vi "Create EQE Data Folder and File Path.vi"(6 "Skip cell?":bool, 7 "Date array":string[](array[string]), 9 "Cell details cluster":T1={"Cell Position"=16, "Cell Label"="", "Pixel to measure"=0, "Area (cm^2)"=0.126, "Variable"="", "Variable value"="", "Scan settings in queue"=0, "Light or dark"="", "Measurement Type"=""} {"Pixel to measure" items=["All", "1", "2", "3", "4", "5", "6", "7", "8"]}, 10 "Experiment Indicator":string, 11 "username":string) -> (1 "EQE data file path string":string, 2 "EQE data file path":path, 3 "EQE Data Output Folder":path)   [LabVIEW 2011]
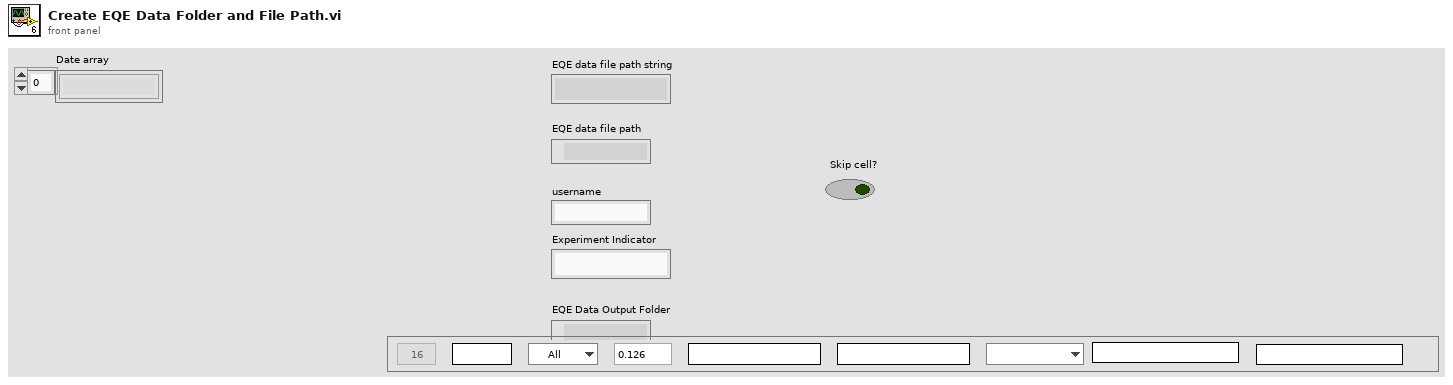
[diagram p1: front panel]
types:
  T1 = cluster{"Cell Position":i32, "Cell Label":string, "Pixel to measure":u16, "Area (cm^2)":dbl, "Variable":string, "Variable value":string, "Scan settings in queue":u16, "Light or dark":string, "Measurement Type":string}
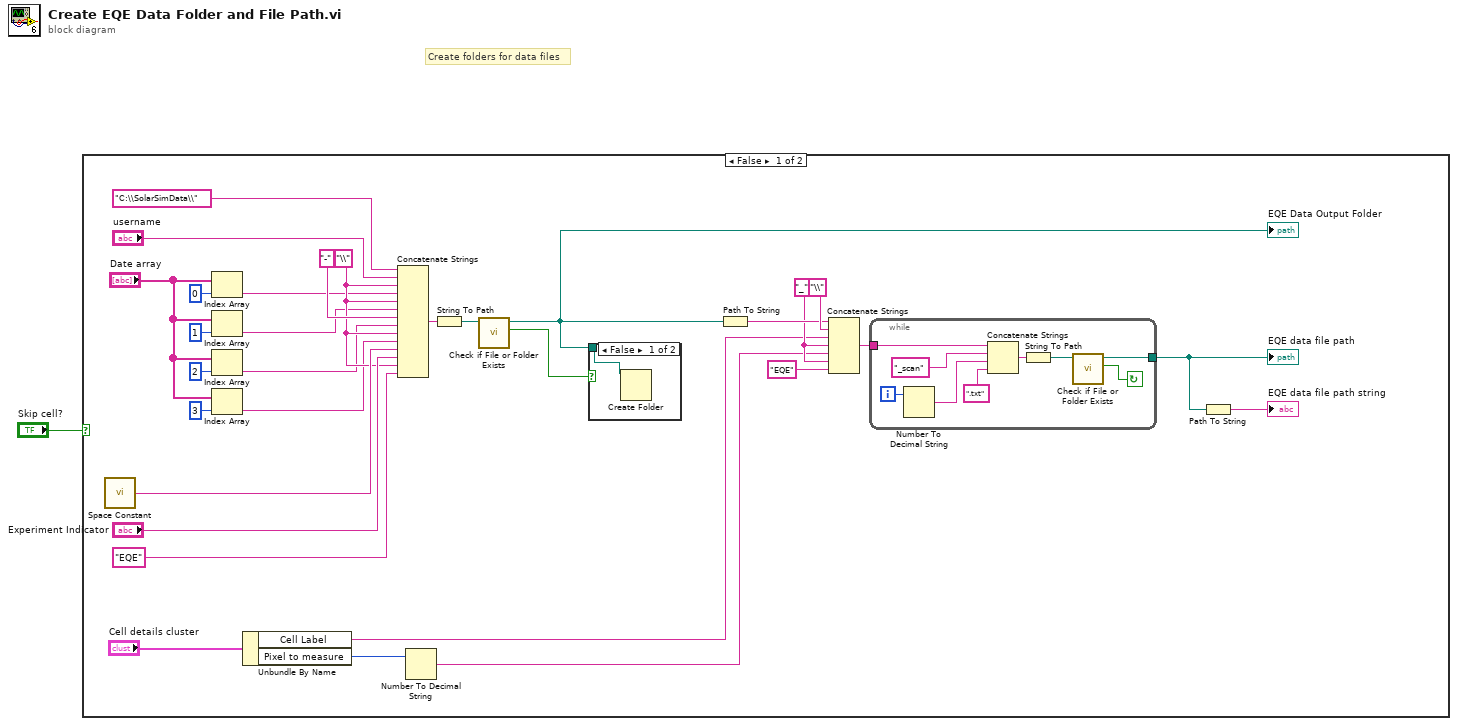
[diagram p0: block diagram]
diagram:
  # "Create folders for data files"
  n1 = case shown="False" "Skip cell?" {
    frame False {
      w19 = "_"
      w24 = "\\"
      n2 = call <vilib>:"Space Constant.vi"() -> ("String"=w26:string)
      n3 = Index Array(array="Date array", index=0) -> (element=w5:string)
      n4 = Index Array(array="Date array", index=1) -> (element=w4:string)
      n5 = Index Array(array="Date array", index=2) -> (element=w3:string)
      n6 = Index Array(array="Date array", index=3) -> (element=w2:string)
      n7 = Unbundle By Name("Cell details cluster") -> ("Cell Label"=w14:string, "Pixel to measure"=w15:u16)
      n8 = Concatenate Strings("C:\\SolarSimData\\", "username", w24, w5, w24, w4, "-", w3, w24, w2, w26, "Experiment Indicator", w24, "EQE") -> (w28:string)
      n9 = Number To Decimal String(number=w15) -> (decimal integer string=w13:string)  [unwired: 1 in]
      n10 = String To Path(string=w28) -> (path=w31:path)
      n11 = call <vilib>:"Check if File or Folder Exists.vi"("path"=w31) -> ("file or folder exists?"=w32:bool, "dup path"=w17:path)  [unwired: 8 in, 1 out]
      "EQE Data Output Folder" <- w17
      n12 = case shown="False" w32 {
        tunnel: w17 -> [w42 _]
        frame False {
          n13 = Create Folder(path (use dialog)=w42) -> ()  [unwired: 2 in, 3 out]
        }
        frame True {
        }
      }
      n14 = Path To String(path=w17) -> (string=w21:string)
      n15 = Concatenate Strings(w21, "\\", w14, w19, w13, w19, "EQE" ("string")) -> (w20:string)
      n16 = while {
        tunnel: w20 -> [w41]
        tunnel: [w33] -> w11
        i -> [w39]
        stop <- w34 continue-if-true
        n17 = Number To Decimal String(number=w39) -> (decimal integer string=w38:string)  [unwired: 1 in]
        n18 = Concatenate Strings(w41, "_scan", w38, ".txt") -> (w35:string)
        n19 = String To Path(string=w35) -> (path=w36:path)
        n20 = call <vilib>:"Check if File or Folder Exists.vi"("path"=w36) -> ("file or folder exists?"=w34:bool, "dup path"=w33:path)  [unwired: 8 in, 1 out]
      }
      "EQE data file path" <- w11
      n21 = Path To String(path=w11) -> (string=→"EQE data file path string":string)
    }
    frame True {
    }
  }
